vi "UT_AddNewStep.vi"   [LabVIEW 2024]
uses:
  <vilib>/addons/_JKI Toolkits/Caraya/classes/Assert/Assert True.vi
  Support/Recipe/Recipe.lvclass
  <vilib>/addons/_JKI Toolkits/Caraya/classes/Test/Test.lvclass
  <vilib>/addons/_JKI Toolkits/Caraya/classes/Assert/Assert.lvclass
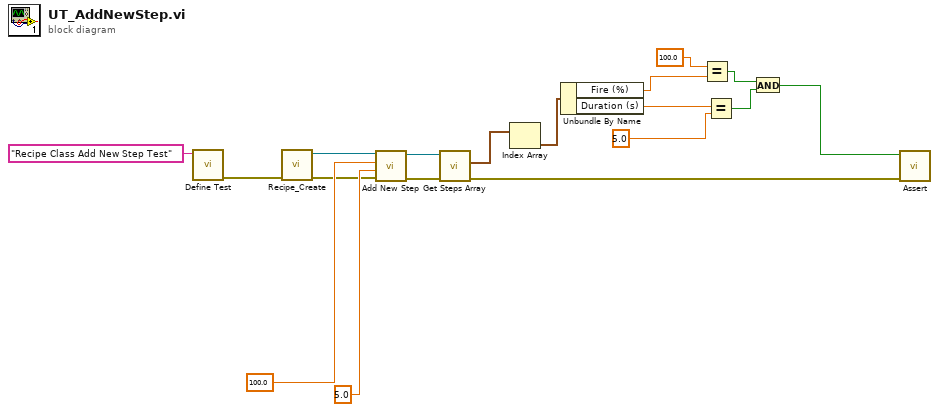
[diagram p0: block diagram]
diagram:
  n1 = call <vilib>:"Define Test.vi"("Label (VI Title)"="Recipe Class Add New Step Test") -> ("error out"=w3:errorcluster)  [unwired: 9 in, 1 out]
  n2 = call "Recipe_Create.vi"("Error In"=w3) -> ("Error Out"=w2:errorcluster, "reference out"=w1:refnum<class "Recipe.lvclass">)  [unwired: 9 in]
  n3 = call-dynamic "Add New Step.vi"("Error In"=w2, "Duration (s)"=5.0, "Fire (%)"=100.0, "reference in"=w1) -> ("Error Out"=w15:errorcluster, "reference out"=w13:refnum<class "Recipe.lvclass">)  [unwired: 6 in]
  n4 = call-dynamic "Get Steps Array.vi"("Error In"=w15, "reference in"=w13) -> ("Error Out"=w14:errorcluster, "Steps"=w12:cluster{"Fire (%)":dbl, "Duration (s)":dbl}[])  [unwired: 7 in, 1 out]
  n5 = Index Array(array=w12) -> (element=w11:cluster{"Fire (%)":dbl, "Duration (s)":dbl})  [unwired: 1 in]
  n6 = Unbundle By Name(w11) -> ("Fire (%)"=w9:dbl, "Duration (s)"=w7:dbl)
  n7 = Equal?(x=100.0 ("Fire (%)"), y=w9) -> (x = y?=w6:bool)
  n8 = Equal?(x=w7, y=5.0 ("Duration (s)")) -> (x = y?=w5:bool)
  n9 = And(x=w6, y=w5) -> (x .and. y?=w4:bool)
  n10 = call-poly <vilib>:"Assert.vi"("error in (no error)"=w14, "True?"=w4) -> ()  [unwired: 8 in, 2 out]
